vi "DjtgDisable.vi"(8 "Error In":errorcluster, 11 "Device Number":u32) -> (0 "Error Out":errorcluster, 3 "Device Number":u32)   [LabVIEW 2011, in "LVH-Adept.lvlib" / "DJTG.lvlib"]
doc: "This function is used to disable and end access to the currently enabled DJTG port on the specified\ninterface handle."
uses:
  DJTG.lvlib
  Private/Type Defs/Error.ctl
  Resources/djtg.dll
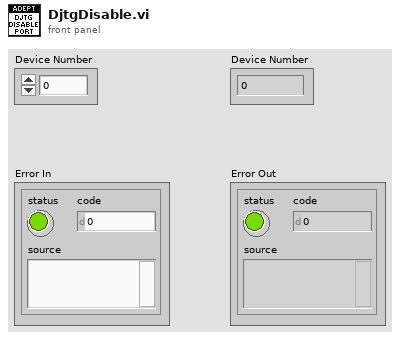
[diagram p1: front panel]
types:
  T1 = typedef "LVH-Adept.lvlib/DJTG.lvlib/Error.ctl" = enum16{"Unknown", "Enable", "PutTmsTdiBits", "GetTdoBits", "Disable", "Close", "Set Aux Reset", "Port Properties", "Get Speed", "Set Speed", "Get Port Count", "Get Batch Properties", "Enable Port", "Set Tmd Tdi Tck", "Get Tms Tdi Tdo Tck", "Put Tdi Bits", "Put Tms Bits", "Clock Tck", "Wait", "Batch", "Flash FPGA"}
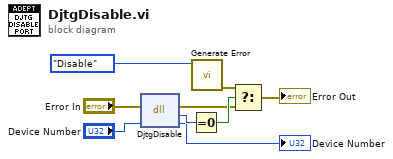
[diagram p0: block diagram]
diagram:
  n1 = dll-call lib="C:/github/labviewhacker/LVH-Adept/LabVIEW/vi.lib/LabVIEW Hacker/Adept/Private/Resources/djtg.dll" fn="DjtgDisable"(error in="Error In", "hif"="Device Number") -> (error out=w4:errorcluster, "Success"=w3:u32, "hif"=→"Device Number":u32)  [unwired: 2 in, 1 out]
  n2 = Equal To 0?(x=w3) -> (x = 0?=w9:bool)
  n3 = call "Generate Error.vi"("DJTG Error"=Error."Disable") -> ("Error Out"=w8:errorcluster)  [unwired: 10 in]
  n4 = Select(t=w8, s=w9, f=w4) -> (s? t:f=→"Error Out":errorcluster)
